vi "Request and Wait for Reply Timeout--error.vi"(11 "Error Message":string) -> (0 "error out":errorcluster)   [LabVIEW 2019, in "FileReader.lvlib"]
doc: "Generate an error for the situation where the Request and Wait for Reply times out.\n_____\nBased on DQMH Project Template 6.1.0.94."
uses:
  FileReader.lvlib
  <vilib>/Utility/error.llb/Error Cluster From Error Code.vi
  <vilib>/ErrorRing/Error Ring.xnode
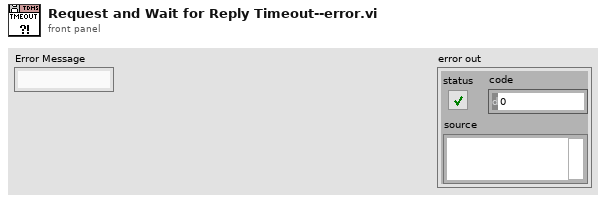
[diagram p1: front panel]
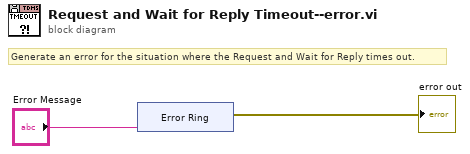
[diagram p0: block diagram]
diagram:
  # "Generate an error for the situation where the Request and Wait for Reply times out."
  n1 = xnode ("Error Ring")("parameter 0"="Error Message") -> ("error out"=→"error out":errorcluster)
